vi "SVM Train NU_SVR.vi"(7 "Options":T1={"cache_size"=200.0, "eps"=0.001, "shrinking"=TRUE, "probability"=FALSE}, 8 "error in (no error)":errorcluster, 9 "Param NU_SVR":T2={"C"=1.0, "nu"=0.5}, 10 "Kernel":T9, 11 "Problem":T8) -> (0 "error out":errorcluster, 3 "Model":T3)   [LabVIEW 2014]
doc: "This function constructs and returns an SVM model according to the given training data and parameters."
uses:
  Controls/Kernel.ctl
  Libsvm Wrapper/Controls/svm_kernel_type.ctl
  Libsvm Wrapper/Controls/svm_problem.ctl
  Libsvm Wrapper/Controls/svm_node.ctl
  Libsvm Wrapper/Controls/svm_model.ctl
  Libsvm Wrapper/Controls/svm_parameter.ctl
  Libsvm Wrapper/Controls/svm_type.ctl
  Controls/Parameters NU_SVR.ctl
  Controls/Options Training.ctl
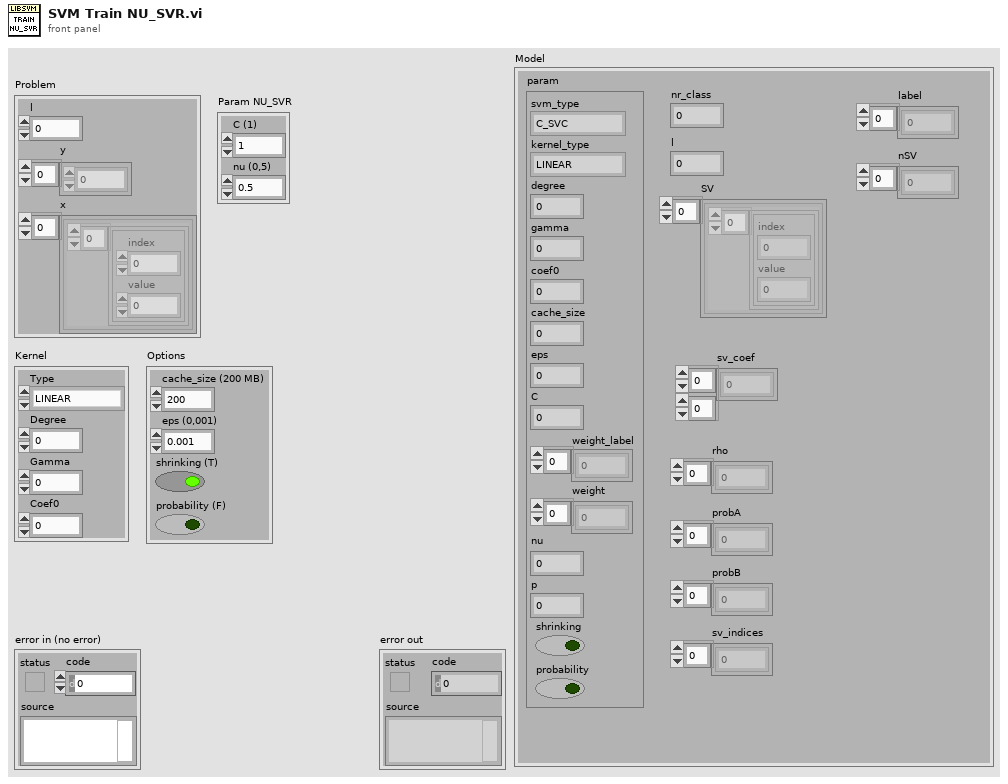
[diagram p1: front panel]
types:
  T1 = typedef "Options Training.ctl" = cluster{"cache_size":dbl, "eps":dbl, "shrinking":bool, "probability":bool}
  T2 = typedef "Parameters NU_SVR.ctl" = cluster{"C":dbl, "nu":dbl}
  T3 = typedef "svm_model.ctl" = cluster{"param":T4, "nr_class":i32, "l":i32, "SV":cluster{"Array":T7[]}[], "sv_coef":dbl[][], "rho":dbl[], "probA":dbl[], "probB":dbl[], "sv_indices":i32[], "label":i32[], "nSV":i32[]}
  T4 = typedef "svm_parameter.ctl" = cluster{"svm_type":T5, "kernel_type":T6, "degree":i32, "gamma":dbl, "coef0":dbl, "cache_size":dbl, "eps":dbl, "C":dbl, "weight_label":i32[], "weight":dbl[], "nu":dbl, "p":dbl, "shrinking":bool, "probability":bool}
  T5 = typedef "svm_type.ctl" = enum32{"C_SVC", "NU_SVC", "ONE_CLASS", "EPSILON_SVR", "NU_SVR"}
  T6 = typedef "svm_kernel_type.ctl" = enum32{"LINEAR", "POLY", "RBF", "SIGMOID", "PRECOMPUTED"}
  T7 = typedef "svm_node.ctl" = cluster{"index":i32, "value":dbl}
  T8 = typedef "svm_problem.ctl" = cluster{"l":i32, "y":dbl[], "x":cluster{T7[]}[]}
  T9 = typedef "Kernel.ctl" = cluster{"Type":T6, "Degree":i32, "Gamma":dbl, "Coef0":dbl}
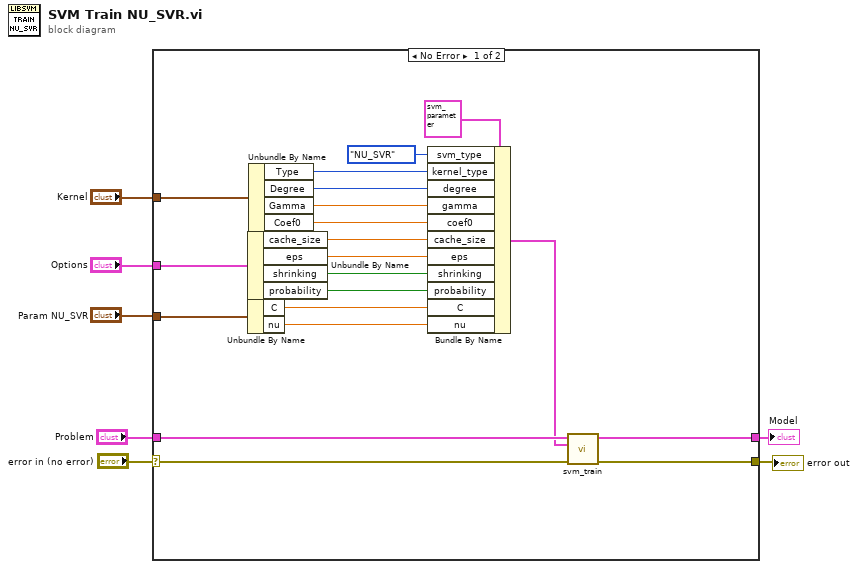
[diagram p0: block diagram]
diagram:
  n1 = case shown="No Error" "error in (no error)" {
    selector: "error in (no error)" -> [w27 w28]
    tunnel: [w26 w28] -> w7
    tunnel: "Problem" -> [w24 _]
    tunnel: "Kernel" -> [w23 _]
    tunnel: [w16 _] -> w3
    tunnel: "Options" -> [w12 _]
    tunnel: "Param NU_SVR" -> [w13 _]
    frame No Error {
      n2 = Unbundle By Name(w12) -> ("cache_size"=w15:dbl, "eps"=w14:dbl, "shrinking"=w11:bool, "probability"=w10:bool)
      n3 = Unbundle By Name(w13) -> ("C"=w9:dbl, "nu"=w8:dbl)
      n4 = Unbundle By Name(w23) -> ("Type"=w22:T6, "Degree"=w21:i32, "Gamma"=w20:dbl, "Coef0"=w19:dbl)
      n5 = Bundle By Name(cluster=T4 {"svm_type"=enum."C_SVC", "kernel_type"=enum."LINEAR", "degree"=0, "gamma"=0.0, "coef0"=0.0, "cache_size"=0.0, "eps"=0.0, "C"=0.0, "weight_label"=[], "weight"=[], "nu"=0.0, "p"=0.0, "shrinking"=FALSE, "probability"=FALSE} ("svm_parameter"), "svm_type"=svm_type."NU_SVR", "kernel_type"=w22, "degree"=w21, "gamma"=w20, "coef0"=w19, "cache_size"=w15, "eps"=w14, "shrinking"=w11, "probability"=w10, "C"=w9, "nu"=w8) -> (w17:T4)
      n6 = call "svm_train.vi"("error in (no error)"=w27, "Parameters"=w17, "Problem"=w24) -> ("error out"=w26:errorcluster, "Model"=w16:T3)  [unwired: 7 in]
    }
    frame Error {
    }
  }
  "error out" <- w7
  "Model" <- w3
